vi "sub_play_DMD_mov.vi"(2 "Exposure (ms)":i32=1000, 3 "SequenceRepeats":i32=1, 4 "binary mov path":path=path "C:/Users/cohen_lab/Desktop/Labview_code/DMD_control/DMD6images.bin") -> (0 "Finished":bool)   [LabVIEW 2012]
uses:
  C:/Program Files/ALP-4.1/ALP-4.1 high-speed API/Samples/alpD41.dll
panel:
  out "Labview":errorcluster
  out "SeqControl3":errorcluster
  out "PicNum":i32
  out "DevFreeErr":i32
  out "SeqFreeErr":i32
  out "ProjWaitErr":i32
  out "ProjStartErr":i32
  out "SeqPutErr":i32
  out "SeqControl1":errorcluster
  out "SeqControl2":errorcluster
  out "SeqTimeErr":i32
  out "ProjControl":errorcluster
  out "SeqAllocErr":i32
  out "DevInq2":errorcluster
  out "DevInq1":errorcluster
  out "DevAllocErr":i32
  in  "Ext. Trig.":bool
  out "DMD Type":string
  out "SequID":u32
  out "DeviceID":u32
  out "SerialNumber":i32
  # "Initialization"
  # "Internal"
  # "External"
  # "0 = no error"
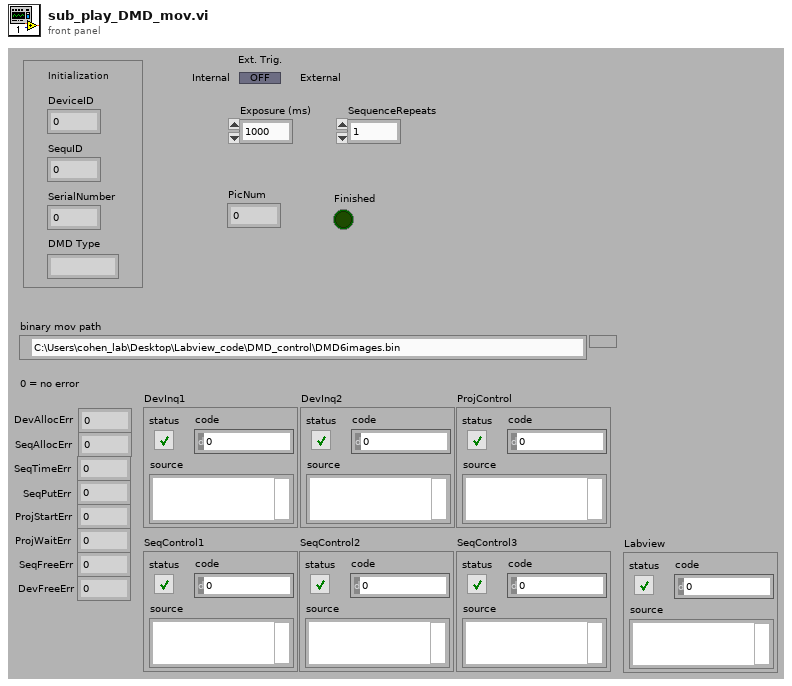
[diagram p1: front panel]
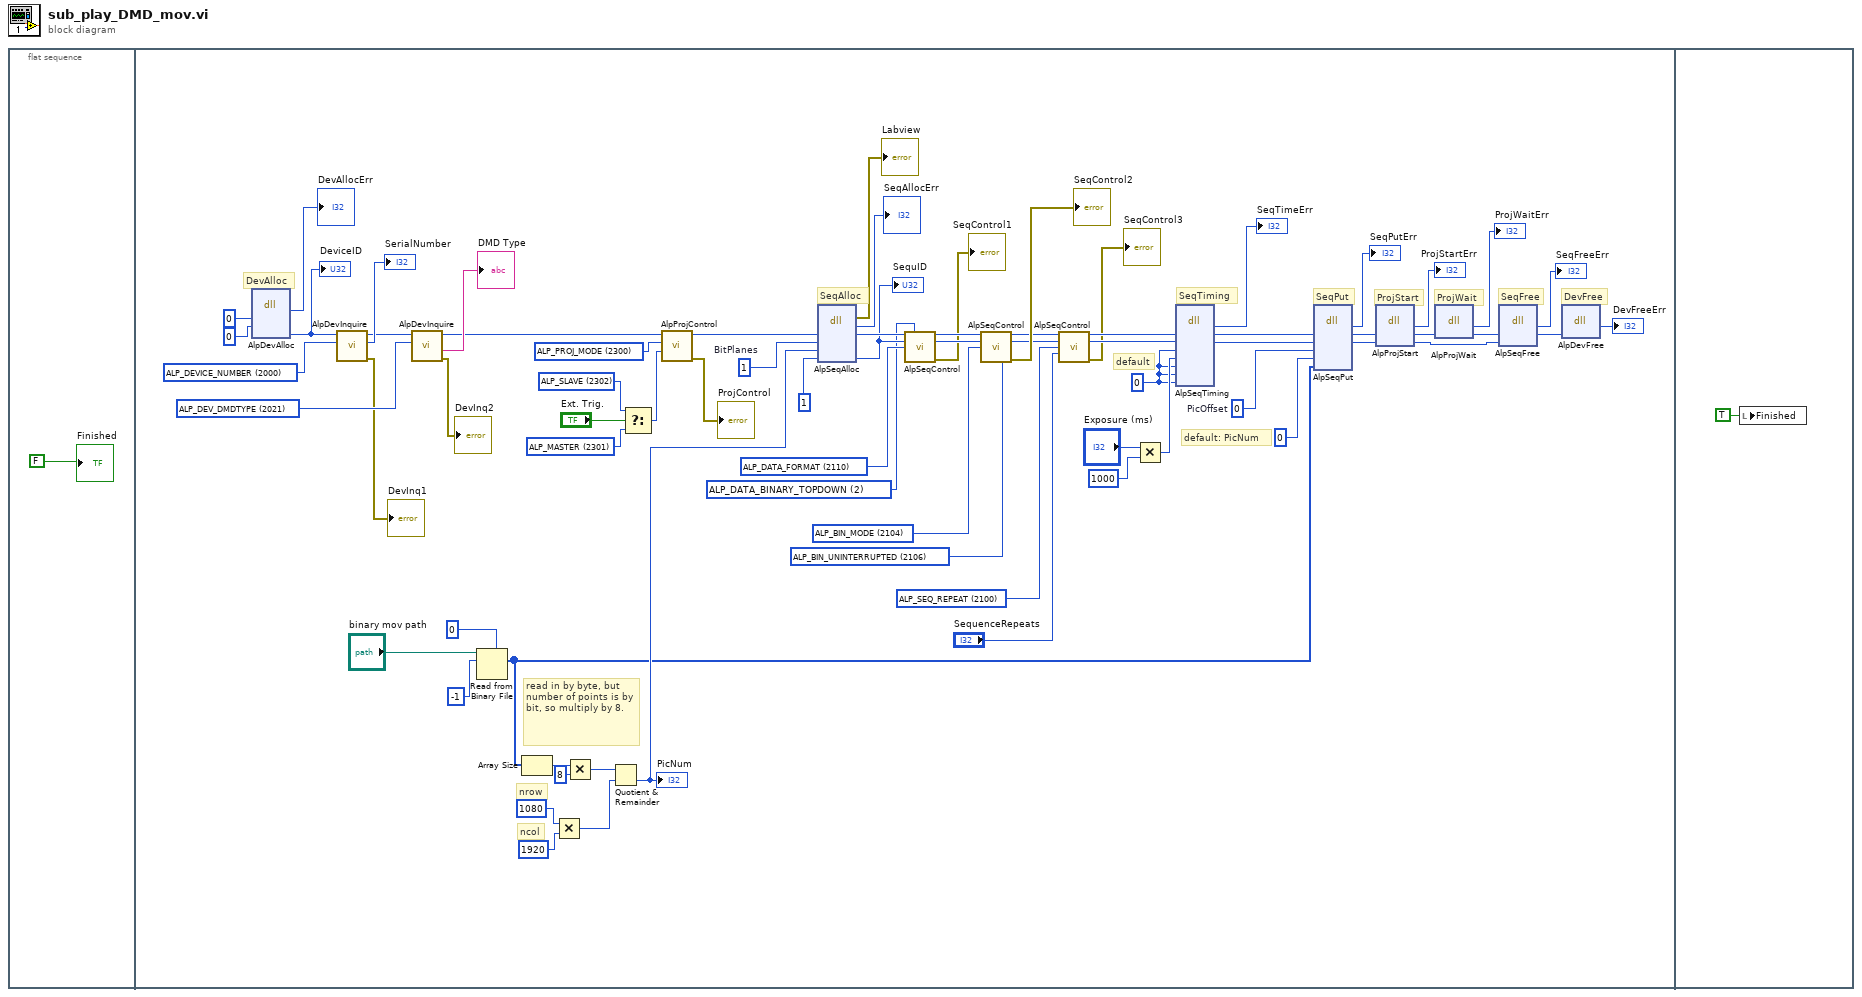
[diagram p0: block diagram]
diagram:
  n1 = flat-sequence {
    frame #0 {
      "Finished" <- FALSE
    }
    frame #1 {
      w7 = 2100 items=["ALP_SEQ_REPEAT"=2100, "ALP_FIRSTFRAME"=2101, "ALP_LASTFRAME"=2102, "ALP_BITNUM"=2103, "ALP_BIN_MODE"=2104, "ALP_DATA_FORMAT"=2110, "ALP_SEQ_PUT_LOCK"=2119] ("ControlType")
      w31 = 2300 items=["ALP_PROJ_MODE"=2300, "ALP_PROJ_INVERSION"=2306, "ALP_PROJ_UPSIDE_DOWN"=2307] ("ControlType")
      w14 = 2301 items=["ALP_MASTER"=2301, "ALP_SLAVE"=2302] ("ProjectorMode")
      w29 = 2302 items=["ALP_MASTER"=2301, "ALP_SLAVE"=2302] ("ProjectorMode")
      w39 = 2106 items=["ALP_BIN_NORMAL"=2105, "ALP_BIN_UNINTERRUPTED"=2106] ("Binary Mode")
      w40 = 2104 items=["ALP_SEQ_REPEAT"=2100, "ALP_FIRSTFRAME"=2101, "ALP_LASTFRAME"=2102, "ALP_BITNUM"=2103, "ALP_BIN_MODE"=2104, "ALP_DATA_FORMAT"=2110, "ALP_SEQ_PUT_LOCK"=2119] ("ControlType")
      w43 = 2 items=["ALP_DATA_MSB_ALIGN", "ALP_DATA_LSB_ALIGN", "ALP_DATA_BINARY_TOPDOWN", "ALP_DATA_BINARY_BOTTOMUP"] ("Data Format")
      w44 = 2110 items=["ALP_SEQ_REPEAT"=2100, "ALP_FIRSTFRAME"=2101, "ALP_LASTFRAME"=2102, "ALP_BITNUM"=2103, "ALP_BIN_MODE"=2104, "ALP_DATA_FORMAT"=2110, "ALP_SEQ_PUT_LOCK"=2119] ("ControlType")
      w50 = 0  # PicOffset
      w51 = 0
      w64 = 2021 items=["ALP_DEVICE_NUMBER"=2000, "ALP_VERSION"=2001, "ALP_DEV_STATE"=2002, "ALP_AVAIL_MEMORY"=2003, "ALP_SYNCH_POLARITY"=2004, "ALP_TRIGGER_EDGE"=2005, "ALP_USB_CONNECTION"=2016, "ALP_DEV_DMDTYPE"=2021, "ALP_DEV_DISPLAY_HEIGHT"=2057, "ALP_DEV_DISPLAY_WIDTH"=2058, "ALP_PWM_LEVEL"=2063, "ALP_DEV_DMD_MODE"=2064] ("InquireType")
      w66 = 2000 items=["ALP_DEVICE_NUMBER"=2000, "ALP_VERSION"=2001, "ALP_DEV_STATE"=2002, "ALP_AVAIL_MEMORY"=2003, "ALP_SYNCH_POLARITY"=2004, "ALP_TRIGGER_EDGE"=2005, "ALP_USB_CONNECTION"=2016, "ALP_DEV_DMDTYPE"=2021, "ALP_DEV_DISPLAY_HEIGHT"=2057, "ALP_DEV_DISPLAY_WIDTH"=2058, "ALP_PWM_LEVEL"=2063, "ALP_DEV_DMD_MODE"=2064] ("InquireType")
      w72 = 1  # BitPlanes
      # "read in by byte, but number of points is by bit, so multiply by 8."
      # "nrow"
      # "ncol"
      # "default: PicNum"
      # "ProjStart"
      # "SeqPut"
      # "ProjWait"
      # "default"
      # "SeqTiming"
      # "DevFree"
      # "SeqFree"
      # "DevAlloc"
      # "SeqAlloc"
      n2 = dll-call lib="C:/Program Files/ALP-4.1/ALP-4.1 high-speed API/Samples/alpD41.dll" fn="AlpDevAlloc"("DeviceNum"=0, "InitFlag"=0) -> ("return type"=→"DevAllocErr":i32, "DeviceIdPtr"=w68:u32)  [unwired: 6 in, 2 out]
      "DeviceID" <- w68
      n3 = call "AlpDevInquire.vi"("InquireType"=w66, "DeviceID"=w68) -> ("Error OUT"=→"DevInq1":errorcluster, "Output Number"=→"SerialNumber":i32, "DeviceIDout"=w65:u32)  [unwired: 6 in, 1 out]
      n4 = call "AlpDevInquire.vi"("InquireType"=w64, "DeviceID"=w65) -> ("Error OUT"=→"DevInq2":errorcluster, "Output Text"=→"DMD Type":string, "DeviceIDout"=w55:u32)  [unwired: 6 in, 1 out]
      n5 = Read from Binary File(5:u8 0, 10:-1 ("count (1)"), 11:"binary mov path") -> (2:w15:u8[])  [unwired: 3 in, 3 out]
      n6 = Array Size(array=w15) -> (size(s)=w12:i32)
      n7 = Multiply(x=1080, y=1920) -> (x*y=w18:i32)
      n8 = Multiply(x=w12, y=8) -> (x*y=w10:i32)
      n9 = Quotient & Remainder(x=w10, y=w18) -> (floor(x/y)=w16:i32)  [unwired: 1 out]
      "PicNum" <- w16
      n10 = Select(t=w29, s="Ext. Trig.", f=w14) -> (s? t:f=w28:i32)
      n11 = call "AlpProjControl.vi"("ProjectorMode"=w28, "ControlType"=w31, "DeviceID"=w55) -> ("Error OUT"=→"ProjControl":errorcluster, "DeviceIDout"=w54:u32)  [unwired: 7 in]
      n12 = dll-call lib="C:/Program Files/ALP-4.1/ALP-4.1 high-speed API/Samples/alpD41.dll" fn="AlpSeqAlloc"("DeviceId"=w54, "BitPlanes"=w72, "PicNum"=w16, "SequenceIdPtr"=u32 1) -> (error out=→"Labview":errorcluster, "return type"=→"SeqAllocErr":i32, "DeviceId"=w46:u32, "SequenceIdPtr"=w45:u32)  [unwired: 5 in, 1 out]
      "SequID" <- w45
      n13 = call "AlpSeqControl.vi"("DeviceID"=w46, "Data Format"=w43, "SequenceID"=w45, "ControlType"=w44) -> ("DeviceIDout"=w42:u32, "SequenceIDout"=w41:u32, "Error OUT"=→"SeqControl1":errorcluster)  [unwired: 9 in]
      n14 = call "AlpSeqControl.vi"("DeviceID"=w42, "SequenceID"=w41, "ControlType"=w40, "Binary Mode"=w39) -> ("DeviceIDout"=w9:u32, "SequenceIDout"=w8:u32, "Error OUT"=→"SeqControl2":errorcluster)  [unwired: 9 in]
      n15 = call "AlpSeqControl.vi"("DeviceID"=w9, "SequenceID"=w8, "ControlType"=w7, "SequenceRepeats"="SequenceRepeats") -> ("DeviceIDout"=w5:u32, "SequenceIDout"=w4:u32, "Error OUT"=→"SeqControl3":errorcluster)  [unwired: 9 in]
      n16 = Multiply(x="Exposure (ms)", y=1000) -> (x*y=w56:i32)
      n17 = dll-call lib="C:/Program Files/ALP-4.1/ALP-4.1 high-speed API/Samples/alpD41.dll" fn="AlpSeqTiming"("DeviceId"=w5, "SequenceId"=w4, "IlluminateTime"=w51, "PictureTime"=w56, "TriggerDelay"=w51, "TriggerPulseWidth"=w51, "VdDelay"=w51) -> ("return type"=→"SeqTimeErr":i32, "DeviceId"=w36:u32, "SequenceId"=w33:u32)  [unwired: 8 in, 2 out]
      n18 = dll-call lib="C:/Program Files/ALP-4.1/ALP-4.1 high-speed API/Samples/alpD41.dll" fn="AlpSeqPut"("DeviceId"=w36, "SequenceId"=w33, "PicOffset"=w50, "PicLoad"=0, "UserArrayPtr"=w15) -> ("return type"=→"SeqPutErr":i32, "DeviceId"=w35:u32, "SequenceId"=w34:u32)  [unwired: 6 in, 2 out]
      n19 = dll-call lib="C:/Program Files/ALP-4.1/ALP-4.1 high-speed API/Samples/alpD41.dll" fn="AlpProjStart" ("alpD40.dll:AlpProjStartCont")("DeviceId"=w35, "SequenceId"=w34) -> ("return type"=→"ProjStartErr":i32, "DeviceId"=w48:u32, "SequenceId"=w47:u32)  [unwired: 3 in, 2 out]
      n20 = dll-call lib="C:/Program Files/ALP-4.1/ALP-4.1 high-speed API/Samples/alpD41.dll" fn="AlpProjWait" ("Knoten zum Aufruf externer Bibliotheken")("DeviceId"=w48) -> ("return type"=→"ProjWaitErr":i32, "DeviceId"=w49:u32)  [unwired: 3 in, 2 out]
      n21 = dll-call lib="C:/Program Files/ALP-4.1/ALP-4.1 high-speed API/Samples/alpD41.dll" fn="AlpSeqFree"("DeviceId"=w49, "SequenceId"=w47) -> ("return type"=→"SeqFreeErr":i32, "DeviceId"=w69:u32)  [unwired: 4 in, 2 out]
      n22 = dll-call lib="C:/Program Files/ALP-4.1/ALP-4.1 high-speed API/Samples/alpD41.dll" fn="AlpDevFree"("DeviceId"=w69) -> ("return type"=→"DevFreeErr":i32)  [unwired: 4 in, 2 out]
    }
    frame #2 {
      n23 = local write "Finished"(TRUE ("Finished")) -> ()
    }
  }
